vi "3_UWV_Read CSV data.vi"() -> ()   [LabVIEW 2015]
uses:
  <vilib>/Utility/file.llb/Read Delimited Spreadsheet (DBL).vi
  <vilib>/Analysis/NI_AALPro.lvlib
panel:
  out "Phase":cluster{dbl, dbl, "all rows":dbl[]}(graph)
  out "Amplitude spectrum":cluster{dbl, dbl, "all rows":dbl[]}(graph)
  out "est frequency peak":dbl format="%0.4f"
  out "Waveform Graph 2":cluster{dbl, dbl, "all rows":dbl[]}(graph)
  in  "stop":bool
  in  "SR":dbl
  in  "number of rows (all:-1)":i32=200000
  out "Waveform Graph":cluster{dbl, dbl, "all rows":dbl[]}(graph)
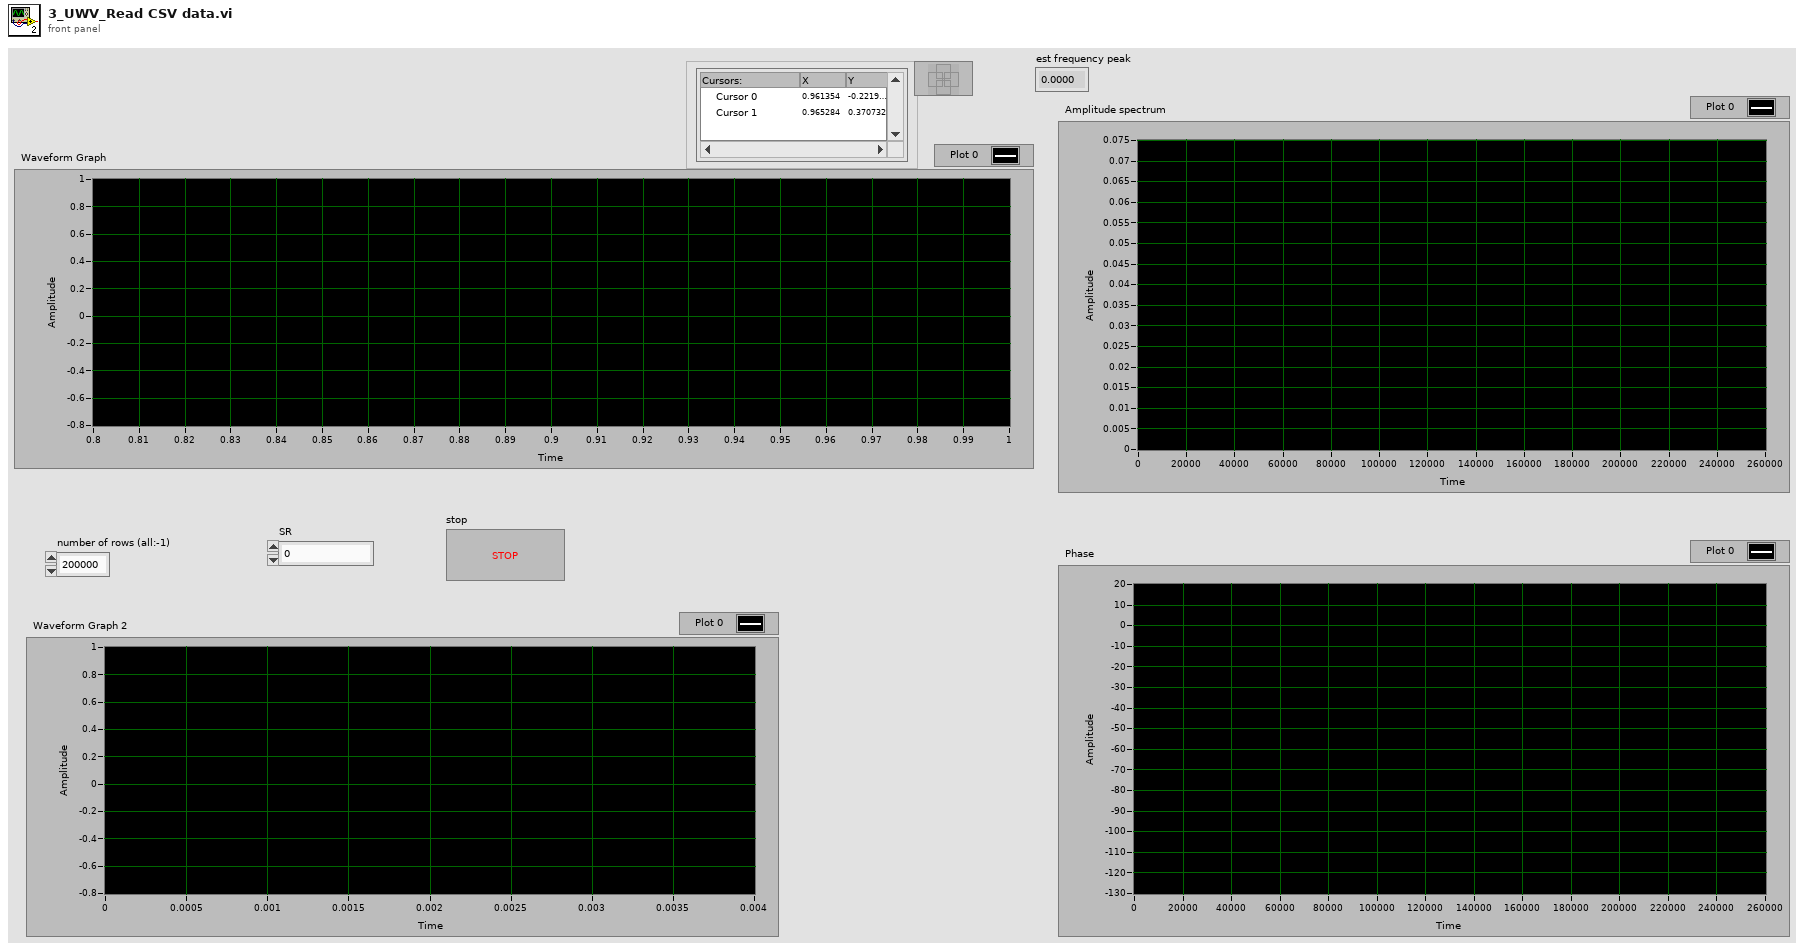
[diagram p1: front panel]
types:
  T1 = cluster{dbl, "df":dbl, "Power Spectrum (V^2 rms)":dbl[]}
  T2 = cluster{dbl, "df":dbl, "Amp Spectrum Phase (radians)":dbl[]}
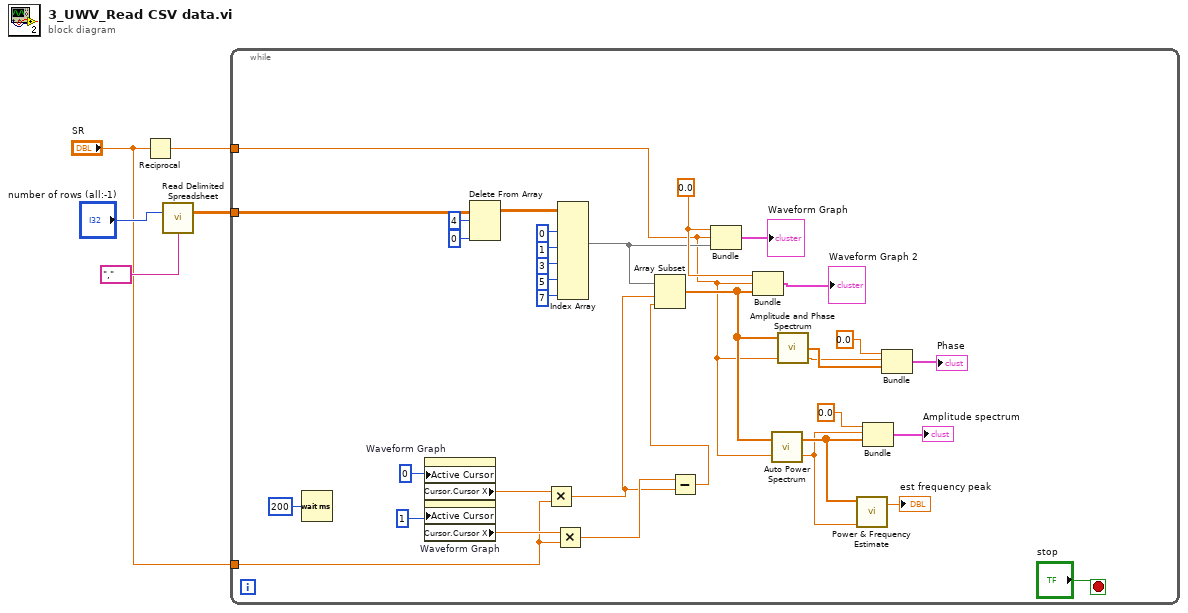
[diagram p0: block diagram]
diagram:
  n1 = Reciprocal(x="SR") -> (1/x=w2:dbl)
  n2 = call-poly <vilib>:"Read Delimited Spreadsheet.vi"("number of rows (all:-1)"="number of rows (all:-1)", "delimiter (\\t)"="," ("delimiter (\\t)")) -> ("all rows"=w4:dbl[][])  [unwired: 8 in, 5 out]
  n3 = while {
    tunnel: w4 -> [w39]
    tunnel: w2 -> [w10]
    tunnel: "SR" -> [w19]
    stop <- "stop" stop-if-true
    w24 = 0.0
    n4 = Wait (ms)(milliseconds to wait=u32 200) -> ()  [unwired: 1 out]
    n5 = property on="Waveform Graph" class="WFGraph (strict)"("Active Cursor"=u32 0) -> ("Cursor.Cursor X"=w21:dbl)  [unwired: 2 in, 2 out]
    n6 = property on="Waveform Graph" class="WFGraph (strict)"("Active Cursor"=u32 1) -> ("Cursor.Cursor X"=w20:dbl)  [unwired: 2 in, 2 out]
    n7 = Delete From Array(array=w39, length=4, index (row)=0) -> (array with subset deleted=w36:dbl[][])  [unwired: 1 in, 1 out]
    n8 = Multiply(x=w21, y=w19) -> (x*y=w17:dbl)
    n9 = Multiply(x=w20, y=w19) -> (x*y=w18:dbl)
    n10 = Index Array(array=w36, index (col) #1=0 ("index (row)"), index (col) #2=1 ("index (row)"), index (col) #3=3 ("index (row)"), index (col) #4=5 ("index (row)"), index (col) #5=7 ("index (row)")) -> (element #2=w22:dbl[])  [unwired: 5 in, 4 out]
    n11 = Subtract(x=w18, y=w17) -> (x-y=w28:dbl)
    n12 = Array Subset(array=w22, index=w17, length=w28) -> (w11:dbl[])
    n13 = Bundle(w24, w10, "all rows"=w22) -> (→"Waveform Graph":cluster{dbl, dbl, "all rows":dbl[]})  [unwired: 1 in]
    n14 = Bundle(w24, w10, w11) -> (→"Waveform Graph 2":cluster{dbl, dbl, dbl[]})  [unwired: 1 in]
    n15 = call <vilib>:"Auto Power Spectrum.vi"("dt"=w10, "Signal (V)"=w11) -> ("df"=w14:dbl, "Power Spectrum (V^2 rms)"=w15:dbl[])
    n16 = call <vilib>:"Amplitude and Phase Spectrum.vi"("dt"=w10, "Signal (V)"=w11) -> ("df"=w7:dbl, "Amp Spectrum Phase (radians)"=w8:dbl[])  [unwired: 1 in, 1 out]
    n17 = call <vilib>:"Power & Frequency Estimate.vi"("df"=w14, "Power Spectrum (V^2 rms)"=w15) -> ("est frequency peak"=→"est frequency peak":dbl)  [unwired: 4 in, 1 out]
    n18 = Bundle(0.0, "df"=w14, "Power Spectrum (V^2 rms)"=w15) -> (→"Amplitude spectrum":T1)  [unwired: 1 in]
    n19 = Bundle(0.0, "df"=w7, "Amp Spectrum Phase (radians)"=w8) -> (→"Phase":T2)  [unwired: 1 in]
  }
